vi "SendToDelete.vi"(8 "error in (no error)":errorcluster, 9 "message value":variant, 10 "Delete?":bool) -> (0 "error out":errorcluster)   [LabVIEW 2015, in "DeleteProcess.lvlib"]
uses:
  DeleteProcess.lvlib
  <vilib>/addons/Qbus/Qbus.lvclass
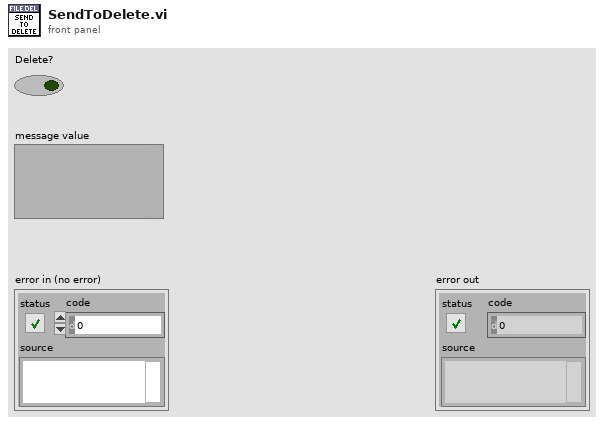
[diagram p1: front panel]
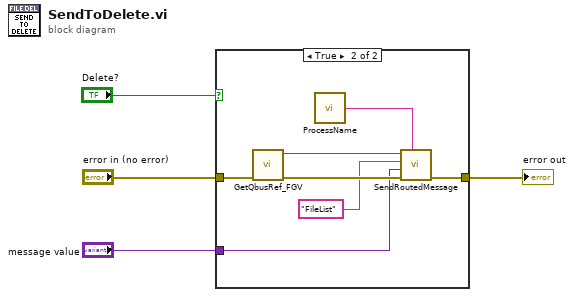
[diagram p0: block diagram]
diagram:
  n1 = case shown="True" "Delete?" {
    tunnel: "error in (no error)" -> [w5 w9]
    tunnel: [w5 w8] -> w3
    tunnel: "message value" -> [_ w6]
    frame False {
    }
    frame True {
      n2 = call <vilib>:"GetQbusRef_FGV.vi"("error in (no error)"=w9) -> ("error out"=w11:errorcluster, "Qbus out"=w12:refnum<class "Qbus.lvclass">)  [unwired: 9 in]
      n3 = call "ProcessName.vi"() -> ("process name"=w10:string)  [unwired: 5 in]
      n4 = call <vilib>:"SendRoutedMessage.vi"("listener process"=w10, "error in (no error)"=w11, "message value"=w6, "message name"="FileList", "Qbus in"=w12) -> ("error in (no error)"=w8:errorcluster)  [unwired: 5 in, 1 out]
    }
  }
  "error out" <- w3
